vi "LabVIEW Measurement UI - Get Parameter.vi"(8 "error in":errorcluster, 11 "Measurement Client Wrapper in":refnum<class "Measurement Client Wrapper.lvclass">) -> (0 "error out":errorcluster, 1 "UI Indicator Details[]":T1[](array[typedef]), 2 "UI Control Details[]":T1[](array[typedef]), 3 "Measurement Client Wrapper":refnum<class "Measurement Client Wrapper.lvclass">)   [LabVIEW 2020, in "Measurement Client Wrapper.lvclass"]
uses:
  Measurement Client Wrapper.lvclass
  Typedefs/Control UI MetaData.ctl
  <vilib>/Utility/Data Type/Type Definitions/Data Type.ctl
  <vilib>/TAF/LabVIEW Measurement Client/RPC Messages/google_protobuf_Field_Kind.ctl
  Measurement Client Wrapper.lvclass/Measurement Client Wrapper.ctl
  <vilib>/Utility/Data Type/NI_Data Type.lvlib
  <vilib>/TAF/LabVIEW Measurement Client/Measurement_client-release.lvlib
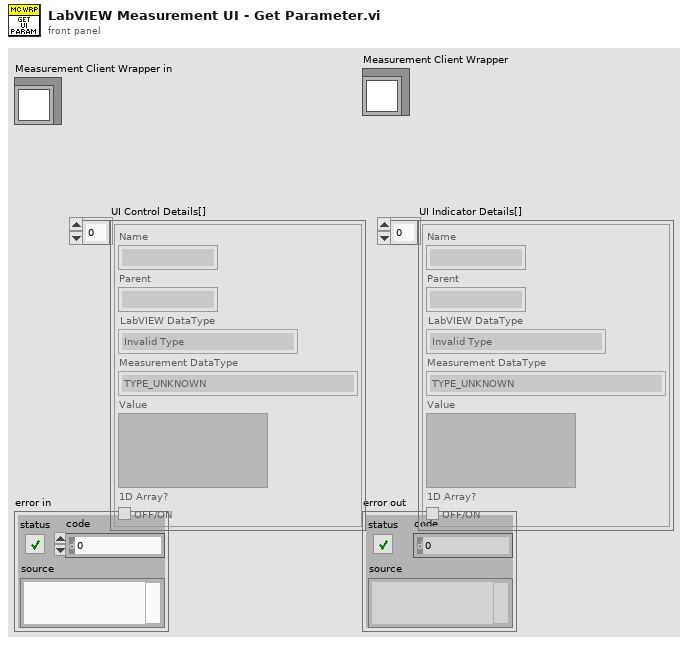
[diagram p1: front panel]
types:
  T1 = typedef "Measurement Client Wrapper.lvclass/Control UI MetaData.ctl" = cluster{"Name":string, "Parent":string, "LabVIEW DataType":T2, "Measurement DataType":T3, "Value":variant, "1D Array?":bool}
  T2 = typedef "NI_Data Type.lvlib/Data Type.ctl" = enum8{"Invalid Type", "Void", "I8", "I16", "I32", "I64", "U8", "U16", "U32", "U64", "Single Float", "Double Float", "Extended Float", "Single Complex", "Double Complex", "Extended Complex", "Enum U8", "Enum U16", "Enum U32", "Enum U64", "Single Float With Unit", "Double Float With Unit", "Extended Float With Unit", "Single Complex with Unit", "Double Complex with Unit", "Extended Complex with Unit", "Boolean", "String", "Path", "Picture", "Tag", "Array", "Cluster", "Variant", "LV Variant", "Waveform", "Timestamp", "Digital Waveform", "Digital Data", "ExpressData", "Refnum", "External Data", "VI", "Poly VI", "LabVIEW Class Instance", "Fixed Point", "Set Collection", "Map Collection"}
  T3 = typedef "Measurement_client-release.lvlib/google_protobuf_Field_Kind.ctl" = enum32{"TYPE_UNKNOWN", "TYPE_DOUBLE", "TYPE_FLOAT", "TYPE_INT64", "TYPE_UINT64", "TYPE_INT32", "TYPE_FIXED64", "TYPE_FIXED32", "TYPE_BOOL", "TYPE_STRING", "TYPE_GROUP", "TYPE_MESSAGE", "TYPE_BYTES", "TYPE_UINT32", "TYPE_ENUM", "TYPE_SFIXED32", "TYPE_SFIXED64", "TYPE_SINT32", "TYPE_SINT64"}
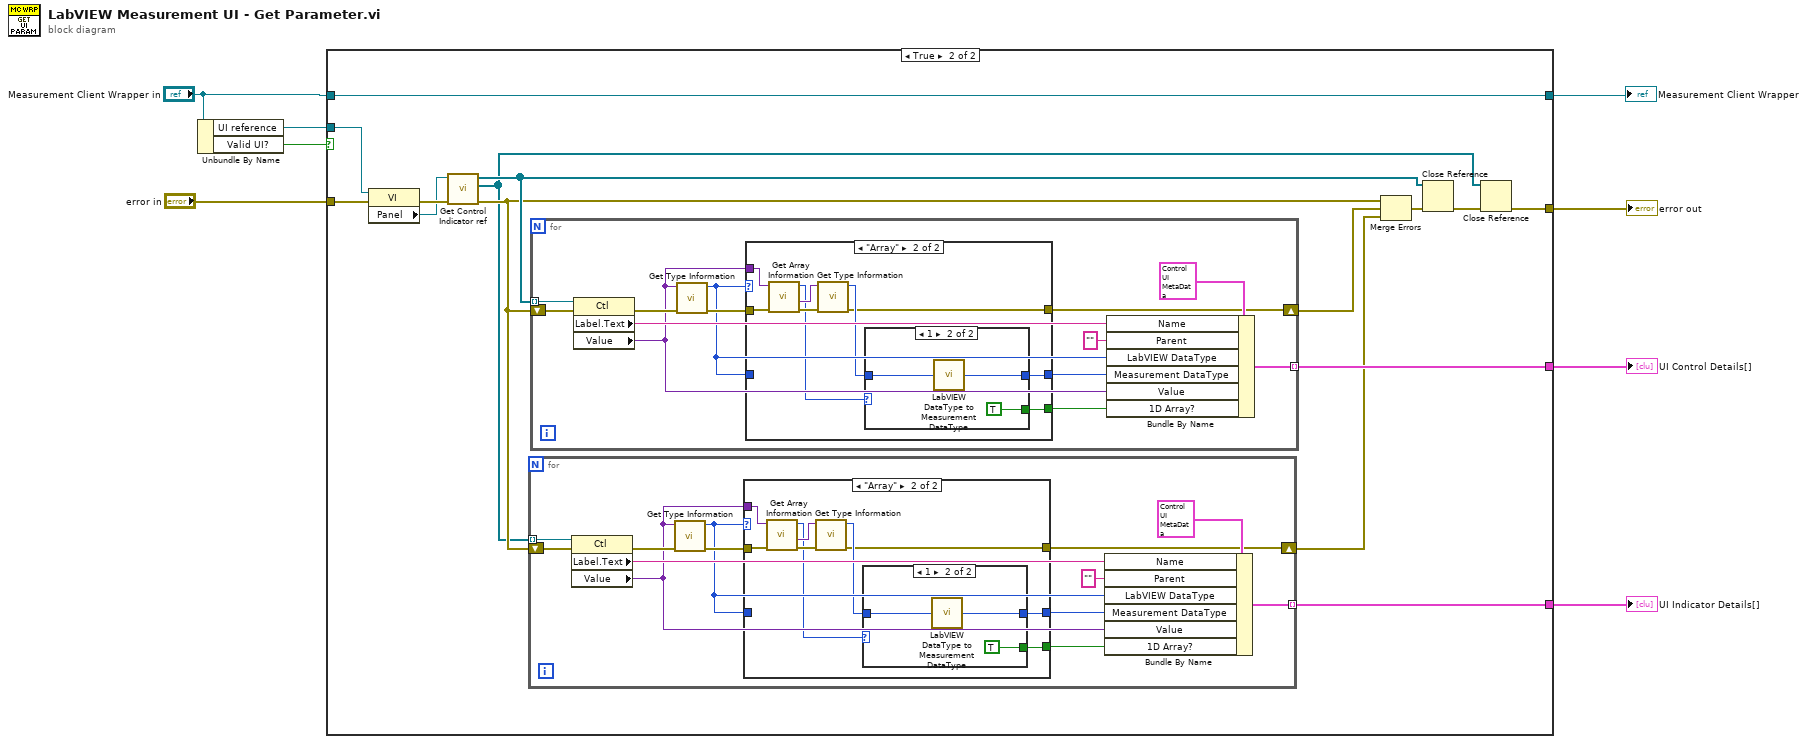
[diagram p0: block diagram]
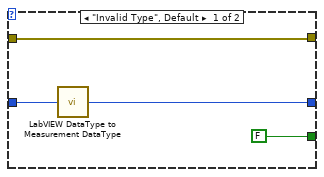
[diagram p3: hidden frame]
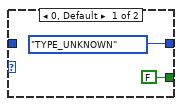
[diagram p4: hidden frame]
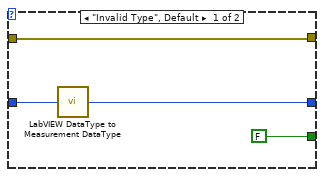
[diagram p5: hidden frame]
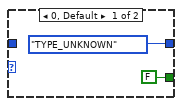
[diagram p6: hidden frame]
diagram:
  n1 = Unbundle By Name("Measurement Client Wrapper in") -> ("UI reference"=w5:refnum<vi>, "Valid UI?"=w3:bool)
  n2 = case shown="True" w3 {
    tunnel: "error in" -> [w9 w25]
    tunnel: [w9 w18] -> w7
    tunnel: [_ w17] -> w6
    tunnel: w5 -> [_ w16]
    tunnel: [_ w13] -> w4
    tunnel: "Measurement Client Wrapper in" -> [w10 w11]
    tunnel: [w10 w11] -> w1
    frame False {
    }
    frame True {
      n3 = property class="VI"(reference=w16, error in=w25) -> (error out=w24:errorcluster, "Panel"=w23:refnum<vi>)  [unwired: 1 out]
      n4 = call "Get Control Indicator ref.vi"("error in"=w24, "panel refnum"=w23) -> ("error out"=w15:errorcluster, "Indicators[]"=w14:refnum<vi>[], "Controls[]"=w20:refnum<vi>[])  [unwired: 7 in]
      n5 = for {
        tunnel: w14 -> [w38] mode=indexing
        shift-right: [w30] -> w12
        shift-left: w15 -> [w37]
        tunnel: [w32] -> w13 mode=indexing
        n6 = property class="Ctl"(reference=w38, error in=w37) -> (error out=w36:errorcluster, "Label.Text"=w34:string, "Value"=w29:variant)  [unwired: 1 out]
        n7 = call <vilib>:"Get Type Information.vi"("error in (no error)"=w36, "variant"=w29) -> ("error out"=w31:errorcluster, "type"=w28:T2)  [unwired: 5 in, 3 out]
        n8 = case shown="\"Array\"" w28 {
          tunnel: w31 -> [w42 w51]
          tunnel: [w42 w45] -> w30
          tunnel: [FALSE w43] -> w26
          tunnel: w29 -> [_ w50]
          tunnel: w28 -> [w40 _]
          tunnel: [w39 w47] -> w27
          frame "Invalid Type", Default {
            n9 = call "LabVIEW DataType to Measurement DataType.vi"("LabVIEW type"=w40) -> ("Measurement DataType"=w39:T3)
          }
          frame "Array" {
            n10 = call <vilib>:"Get Array Information.vi"("error in (no error)"=w51, "variant"=w50) -> ("error out"=w46:errorcluster, "array element data type"=w49:variant, "number of dimensions"=w44:i32)  [unwired: 6 in, 1 out]
            n11 = call <vilib>:"Get Type Information.vi"("error in (no error)"=w46, "variant"=w49) -> ("error out"=w45:errorcluster, "type"=w48:T2)  [unwired: 5 in, 3 out]
            n12 = case shown="1" w44 {
              tunnel: w48 -> [_ w56]
              tunnel: [google_protobuf_Field_Kind."TYPE_UNKNOWN" ("Measurement DataType") w55] -> w47
              tunnel: [FALSE TRUE] -> w43
              frame 0, Default {
              }
              frame 1 {
                n13 = call "LabVIEW DataType to Measurement DataType.vi"("LabVIEW type"=w56) -> ("Measurement DataType"=w55:T3)
              }
            }
          }
        }
        n14 = Bundle By Name(cluster=T1 {"Name"="", "Parent"="", "LabVIEW DataType"=enum."Invalid Type", "Measurement DataType"=enum."TYPE_UNKNOWN", "Value"=variant, "1D Array?"=FALSE} ("Control Details"), "Name"=w34, "Parent"="", "LabVIEW DataType"=w28, "Measurement DataType"=w27, "Value"=w29, "1D Array?"=w26) -> (w32:T1)
      }
      n15 = for {
        tunnel: w20 -> [w69] mode=indexing
        shift-right: [w61] -> w21
        shift-left: w15 -> [w68]
        tunnel: [w63] -> w17 mode=indexing
        n16 = property class="Ctl"(reference=w69, error in=w68) -> (error out=w67:errorcluster, "Label.Text"=w65:string, "Value"=w60:variant)  [unwired: 1 out]
        n17 = call <vilib>:"Get Type Information.vi"("error in (no error)"=w67, "variant"=w60) -> ("error out"=w62:errorcluster, "type"=w59:T2)  [unwired: 5 in, 3 out]
        n18 = case shown="\"Array\"" w59 {
          tunnel: w62 -> [w73 w82]
          tunnel: [w73 w76] -> w61
          tunnel: [FALSE w74] -> w57
          tunnel: w60 -> [_ w81]
          tunnel: w59 -> [w71 _]
          tunnel: [w70 w78] -> w58
          frame "Invalid Type", Default {
            n19 = call "LabVIEW DataType to Measurement DataType.vi"("LabVIEW type"=w71) -> ("Measurement DataType"=w70:T3)
          }
          frame "Array" {
            n20 = call <vilib>:"Get Array Information.vi"("error in (no error)"=w82, "variant"=w81) -> ("error out"=w77:errorcluster, "array element data type"=w80:variant, "number of dimensions"=w75:i32)  [unwired: 6 in, 1 out]
            n21 = call <vilib>:"Get Type Information.vi"("error in (no error)"=w77, "variant"=w80) -> ("error out"=w76:errorcluster, "type"=w79:T2)  [unwired: 5 in, 3 out]
            n22 = case shown="1" w75 {
              tunnel: w79 -> [_ w87]
              tunnel: [google_protobuf_Field_Kind."TYPE_UNKNOWN" ("Measurement DataType") w86] -> w78
              tunnel: [FALSE TRUE] -> w74
              frame 0, Default {
              }
              frame 1 {
                n23 = call "LabVIEW DataType to Measurement DataType.vi"("LabVIEW type"=w87) -> ("Measurement DataType"=w86:T3)
              }
            }
          }
        }
        n24 = Bundle By Name(cluster=T1 {"Name"="", "Parent"="", "LabVIEW DataType"=enum."Invalid Type", "Measurement DataType"=enum."TYPE_UNKNOWN", "Value"=variant, "1D Array?"=FALSE} ("Control Details"), "Name"=w65, "Parent"="", "LabVIEW DataType"=w59, "Measurement DataType"=w58, "Value"=w60, "1D Array?"=w57) -> (w63:T1)
      }
      n25 = Merge Errors(w15, w21, w12) -> (w22:errorcluster)
      n26 = Close Reference(reference=w20, error in (no error)=w22) -> (error out=w19:errorcluster)
      n27 = Close Reference(reference=w14, error in (no error)=w19) -> (error out=w18:errorcluster)
    }
  }
  "error out" <- w7
  "UI Control Details[]" <- w6
  "UI Indicator Details[]" <- w4
  "Measurement Client Wrapper" <- w1
